vi "Set Input Channel Section.vi"(8 "error in (no error)":errorcluster, 10 "Input Channel Parameters":T1={"AI MaxV"=0.0, "AI MinV"=0.0, "AI Sample Rate"=0.0, "Input Configuration"=10083} {"Input Configuration" items=["RSE"=10083, "NRSE"=10078, "Differential"=10106]}, 11 "Ref in":T2 format="%.0x") -> (0 "error out":errorcluster, 3 "Ref out":T2 format="%.0x")   [LabVIEW 2021, in "DAQ Analog InOut System Explorer.lvlib"]
uses:
  <vilib>/NI VeriStand/Custom Device API/Custom Device Item Ref.ctl
  Types/Input Channel Parameters.ctl
  Shared/Constants.vi
  <vilib>/NI VeriStand/Custom Device API/Set Item Property (Variant).vi
  DAQ Analog InOut System Explorer.lvlib
  <vilib>/NI VeriStand/Custom Device API/Custom Device API.lvlib
  Shared/DAQ Analog InOut Shared.lvlib
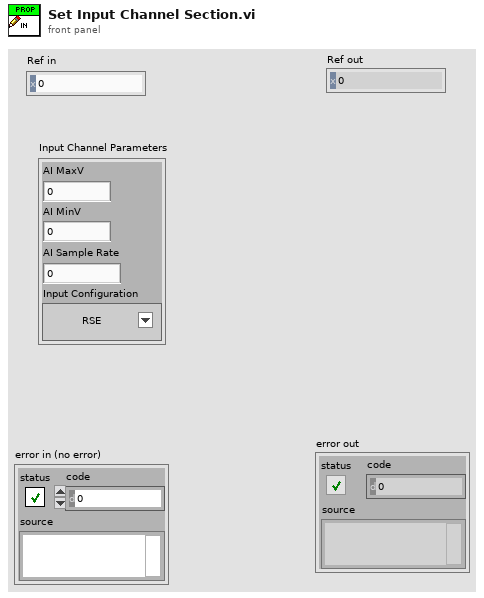
[diagram p1: front panel]
types:
  T1 = typedef "DAQ Analog InOut System Explorer.lvlib/Input Channel Parameters.ctl" = cluster{"AI MaxV":dbl, "AI MinV":dbl, "AI Sample Rate":dbl, "Input Configuration":u16}
  T2 = typedef "Custom Device API.lvlib/Custom Device Item Ref.ctl" = u64
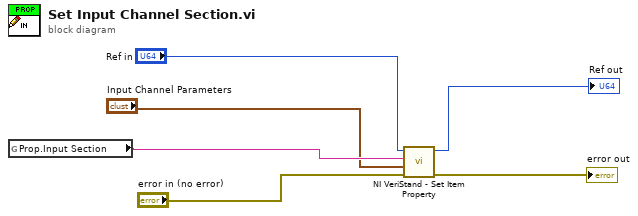
[diagram p0: block diagram]
diagram:
  n1 = global read "Constants.vi" "Prop.Input Section"() -> (w2:string)
  n2 = call-poly <vilib>:"NI VeriStand - Set Item Property.vi"("error in (no error)"="error in (no error)", "Value"="Input Channel Parameters", "Property Name"=w2, "Item Ref in"="Ref in") -> ("error out"=→"error out":errorcluster, "Item Ref out"=→"Ref out":T2)  [unwired: 5 in, 1 out]
